vi "Open Session with Retires and Error Clearing.vi"(8 "error in":errorcluster, 9 "\"Wait for Session\" Timeout (3000 ms)":u32=3000, 10 "Number of \"Open Session\" Retry Attempts (3)":i32=3, 11 "VISA Resource Name":refnum<visa-resource-name>) -> (0 "error out":errorcluster, 1 "Elapsed Time (ms)":u32, 2 "IN_SESSION":bool, 3 "dup VISA Resource Name":refnum<visa-resource-name>)   [LabVIEW 2020]
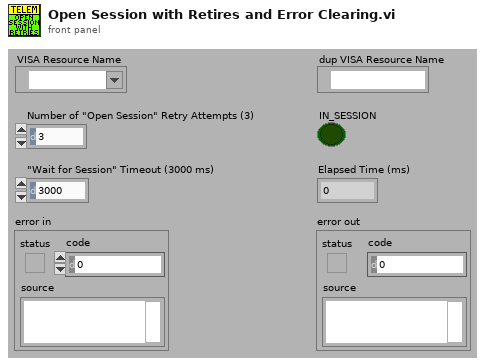
[diagram p1: front panel]
types:
  T1 = enum16{"Get Device Type", "Get Device Name", "Get Device Version", "Get Device Error"}
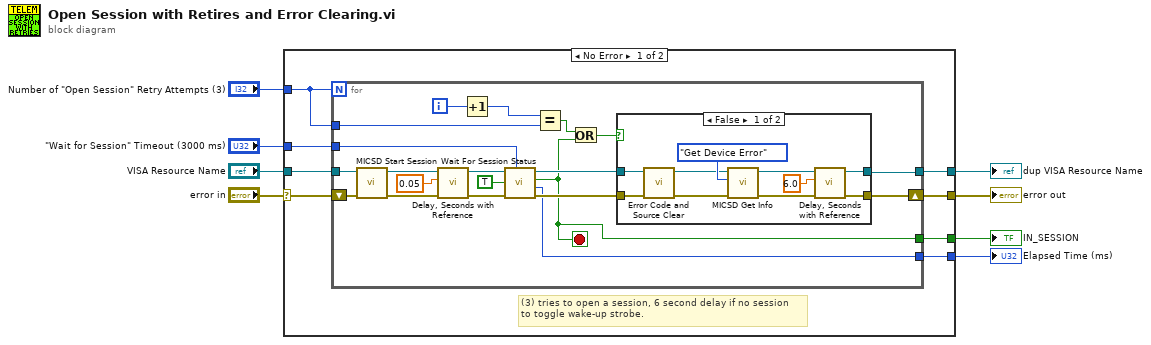
[diagram p0: block diagram]
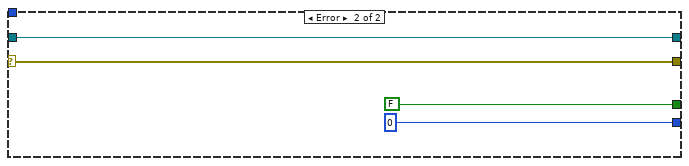
[diagram p3: hidden frame]
diagram:
  n1 = case shown="No Error" "error in" {
    selector: "error in" -> [w13 w50]
    tunnel: [w16 w51] -> w8
    tunnel: [w15 w50] -> w7
    tunnel: "VISA Resource Name" -> [w14 w51]
    tunnel: "\"Wait for Session\" Timeout (3000 ms)" -> [w12 _]
    tunnel: "Number of \"Open Session\" Retry Attempts (3)" -> [w11 _]
    tunnel: [w10 FALSE ("IN_SESSION")] -> w2
    tunnel: [w9 u32 0 ("Elapsed Time (ms)")] -> w1
    frame No Error {
      # "(3) tries to open a session, 6 second delay if no session\nto toggle wake-up strobe."
      n2 = for {
        N: w11 -> [_]
        tunnel: w14 -> [w35]
        tunnel: [w31] -> w16
        shift-right: [w30] -> w15
        shift-left: w13 -> [w34]
        tunnel: w12 -> [w29]
        tunnel: w11 -> [w28]
        tunnel: [w25] -> w10
        tunnel: [w24] -> w9
        i -> [w23]
        stop <- w25 stop-if-true
        n3 = call "MICSD Start Session.vi"("error in (no error)"=w34, "VISA Resource Name"=w35) -> ("error out"=w19:errorcluster, "dup VISA Resource Name"=w21:refnum<visa-resource-name>)  [unwired: 8 in]
        n4 = call "Delay, Seconds with Reference.vi"("error in"=w19, "delay"=dbl[unit] 0.05, "VISA resource"=w21) -> ("error out"=w18:errorcluster, "VISA resource dup"=w20:refnum<visa-resource-name>)  [unwired: 3 in, 1 out]
        n5 = Increment(x=w23) -> (x+1=w22:i32)
        n6 = call "Wait For Session Status.vi"("Timeout (3000 ms)"=w29, "error in (no error)"=w18, "IN_SESSION State (T)"=TRUE, "VISA Resource Name"=w20) -> ("error out"=w33:errorcluster, "Elapsed Time (ms)"=w24:u32, "IN_SESSION"=w25:bool, "dup VISA Resource Name"=w32:refnum<visa-resource-name>)  [unwired: 4 in]
        n7 = Equal?(x=w22, y=w28) -> (x = y?=w26:bool)
        n8 = Or(x=w26, y=w25) -> (x .or. y?=w27:bool)
        n9 = case shown="False" w27 {
          tunnel: w33 -> [w43 w46]
          tunnel: w32 -> [w40 w47]
          tunnel: [w44 w47] -> w31
          tunnel: [w42 w46] -> w30
          frame False {
            n10 = call "Error Code and Source Clear.vi"("error in"=w43) -> ("error out"=w38:errorcluster)  [unwired: 8 in]
            n11 = call "MICSD Get Info.vi"("error in (no error)"=w38, "Command"=T1."Get Device Error", "VISA Resource Name"=w40) -> ("error out"=w37:errorcluster, "dup VISA Resource Name"=w39:refnum<visa-resource-name>)  [unwired: 6 in, 1 out]
            n12 = call "Delay, Seconds with Reference.vi"("error in"=w37, "delay"=dbl[unit] 6.0, "VISA resource"=w39) -> ("error out"=w42:errorcluster, "VISA resource dup"=w44:refnum<visa-resource-name>)  [unwired: 3 in, 1 out]
          }
          frame True {
          }
        }
      }
    }
    frame Error {
    }
  }
  "dup VISA Resource Name" <- w8
  "error out" <- w7
  "IN_SESSION" <- w2
  "Elapsed Time (ms)" <- w1
